vi "Close.vi"(8 "error in (no error)":errorcluster, 11 "VISA resource name in":refnum<visa-resource-name>) -> (0 "error out":errorcluster)   [LabVIEW 2021, in "UART.lvlib"]
uses:
  <vilib>/myRIO/Instrument Drivers/Onboard IO/UART/UART.lvlib
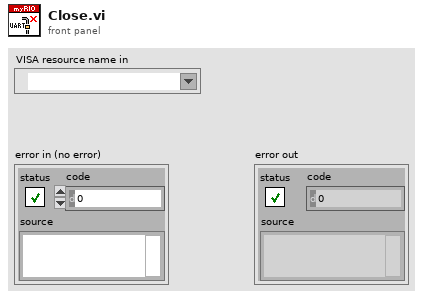
[diagram p1: front panel]
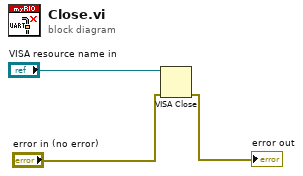
[diagram p0: block diagram]
diagram:
  n1 = VISA Close(VISA resource name="VISA resource name in", error in (no error)="error in (no error)") -> (error out=→"error out":errorcluster)
